vi "SSH_ReadWrite.vi"(6 "Timeout (ms)":u32, 8 "error in (no error)":errorcluster, 9 "Wait for":string, 10 "To Send":string, 11 "Python in":cluster{"Python":refnum<k35>, "py file":path}) -> (0 "error out":errorcluster, 1 "Console":string)   [LabVIEW 2020]
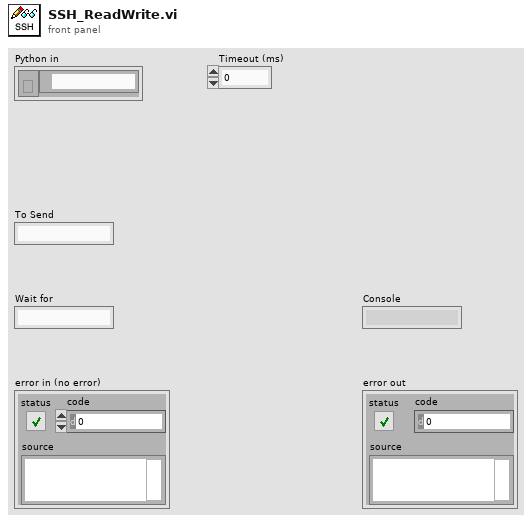
[diagram p1: front panel]
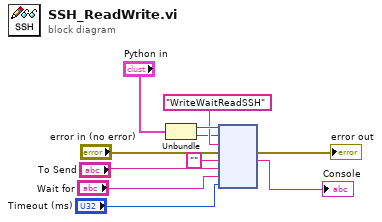
[diagram p0: block diagram]
diagram:
  n1 = Unbundle("Python in") -> ("Python"=w11:refnum<k35>, "py file"=w2:path)
  n2 = node(w11, w2, "WriteWaitReadSSH" ("function name"), "error in (no error)", "" ("function name"), "To Send", "Wait for", "Timeout (ms)") -> (→"error out":errorcluster, →"Console":string)  [unwired: 3 in, 3 out]
